vi "ma_SML RT Baseband Zoom FFT (complex input).vi"(0 "x [V]":cdb[](array[numeric]) format="%.2f", 5 "zoom settings":T2={"zoom"=1, "stop band attenuation"=enum."120 dB", "alias protect in final transition"=FALSE, "oversampling ratio"=1.0} {"oversampling ratio" format="%.2f"; "zoom" min=0}, 7 "FFT settings":T3={"window"=1, "Window Size"=1024, "FFT Size"=1024, "%overlap"=0.0} {"window" items=["Rectangle"=0, "Hanning"=1, "Hamming"=2, "Blackman-Harris"=3, "Exact Blackman"=4, "Blackman"=5, "Flat Top"=6, "4 Term B-Harris "=7, "7 Term B-Harris"=8, "Low Sidelobe"=9, "Blackman Nuttall"=11, "Triangle"=30, "Bartlett-Hanning"=31, "Bohman"=32, "Parzen"=33, "Welch"=34, "Kaiser"=60, "Dolph-Chebyshev"=61, "Gaussian"=62]; "%overlap" min=0.0 max=100.0 format="%.2f"}, 11 "error in (no error)":errorcluster, 12 "reset?":bool) -> (4 "FFT{X} [Vrms]":cdb[](array[numeric]) format="%.2f", 6 "time data":cdb[](array[numeric]) format="%.2f", 8 "spectral info":T1 {"window" items=["Rectangle"=0, "Hanning"=1, "Hamming"=2, "Blackman-Harris"=3, "Exact Blackman"=4, "Blackman"=5, "Flat Top"=6, "4 Term B-Harris "=7, "7 Term B-Harris"=8, "Low Sidelobe"=9, "Blackman Nuttall"=11, "Triangle"=30, "Bartlett-Hanning"=31, "Bohman"=32, "Parzen"=33, "Welch"=34, "Kaiser"=60, "Dolph-Chebyshev"=61, "Gaussian"=62]}, 10 "spectrum ready?":bool, 14 "filter transition length":i32=1 min=0, 15 "error out":errorcluster)   [LabVIEW 2020, in "NI_MAPro.lvlib"]
uses:
  NI_MAPro.lvlib
  ma_sml_Spectral Info.ctl
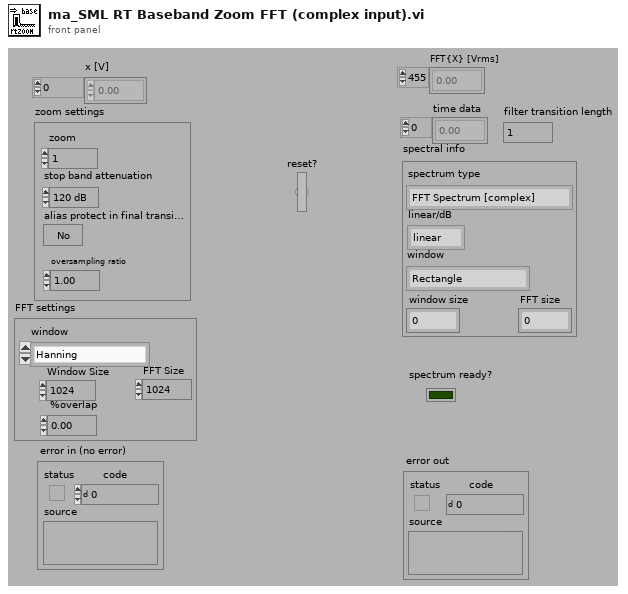
[diagram p1: front panel]
types:
  T1 = typedef "NI_MAPro.lvlib/ma_sml_Spectral Info.ctl" = cluster{"spectrum type":enum16{"FFT Spectrum [complex]", "Amplitude [Magnitude]", "Power [Magnitude^2]", "Cross Spectrum [complex]", "Frequency Response [Complex]"}, "linear/dB":enum16{"linear", "dB"}, "window":u16, "window size":i32, "FFT size":i32}
  T2 = cluster{"zoom":i32, "stop band attenuation":enum16{"84 dB", "96 dB", "120 dB"}, "alias protect in final transition":bool, "oversampling ratio":dbl}
  T3 = cluster{"window":u16, "Window Size":i32, "FFT Size":i32, "%overlap":dbl}
  T4 = cluster{"zoom":bool, "stop band attenuation":bool, "alias protect in final transition":bool, "oversampling ratio":bool}
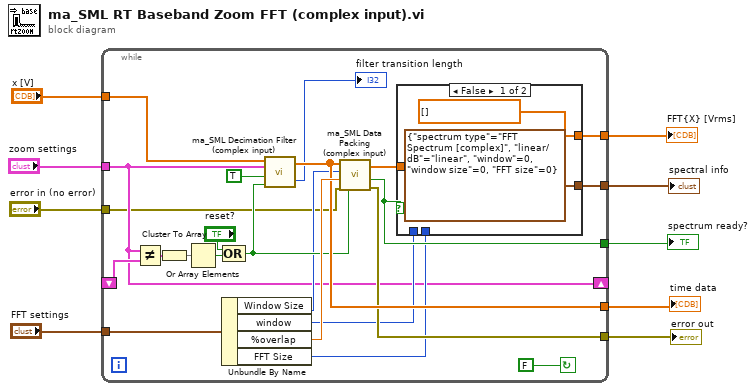
[diagram p0: block diagram]
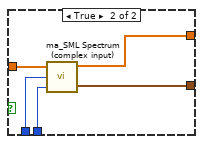
[diagram p2: hidden frame]
diagram:
  n1 = while {
    tunnel: "FFT settings" -> [w10]
    tunnel: "error in (no error)" -> [w11]
    tunnel: [w12] -> w3
    tunnel: "x [V]" -> [w13]
    tunnel: "zoom settings" -> [w14]
    tunnel: [w22] -> w6
    tunnel: [w23] -> w7
    tunnel: [w24] -> w8
    shift-left: _ -> [w25]
    shift-right: [w14] -> _
    tunnel: [w32] -> w9
    stop <- FALSE continue-if-true
    n2 = Not Equal?(x=w14, y=w25) -> (x != y?=w28:T4)
    n3 = Cluster To Array(cluster=w28) -> (array=w27:bool[])
    n4 = Or Array Elements(Boolean array=w27) -> (logical OR=w30:bool)
    n5 = Unbundle By Name(w10) -> ("Window Size"=w19:i32, "window"=w18:u16, "%overlap"=w29:dbl, "FFT Size"=w17:i32)
    n6 = Compound Arithmetic op=OR("reset?", w30) -> (w21:bool)
    n7 = call "ma_SML Decimation Filter (complex input).vi"("reset?"=w21, "truncate transition?"=TRUE ("Truncate initial filter Transition"), "decimation setting"=w14, "x"=w13) -> ("initial cutoff length"=→"filter transition length":i32, "y"=w24:cdb[])
    n8 = call "ma_SML Data Packing (complex input).vi"("reset?"=w21, "error in (no error)"=w11, "%overlap"=w29, "size"=w19, "x"=w24) -> ("error out"=w23:errorcluster, "data ready?"=w32:bool, "y"=w31:cdb[])  [unwired: 4 in]
    n9 = case shown="False" w32 {
      tunnel: [cdb[] [] ("FFT{x} [Vrms]") w39] -> w22
      tunnel: w31 -> [_ w37]
      tunnel: w18 -> [_ w38]
      tunnel: w17 -> [_ w36]
      tunnel: [T1 {"spectrum type"=enum."FFT Spectrum [complex]", "linear/dB"=enum."linear", "window"=0, "window size"=0, "FFT size"=0} ("spectral info") w35] -> w12
      frame False {
      }
      frame True {
        n10 = call "ma_SML Spectrum (complex input).vi"("FFT size"=w36, "window"=w38, "x [V]"=w37) -> ("spectral info"=w35:T1, "FFT{x} [Vrms]"=w39:cdb[])
      }
    }
  }
  "spectrum ready?" <- w9
  "FFT{X} [Vrms]" <- w6
  "time data" <- w8
  "error out" <- w7
  "spectral info" <- w3
